vi "add_word.vi"(11 "子数组":u8[](array[numeric])) -> (3 "校验通过":bool)   [LabVIEW 2012]
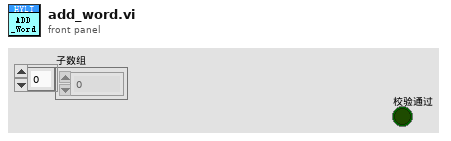
[diagram p1: front panel]
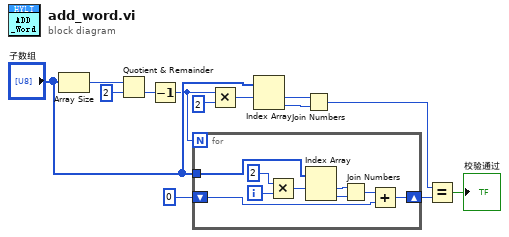
[diagram p0: block diagram]
diagram:
  n1 = Array Size(array="子数组") -> (size(s)=w11:i32)
  n2 = Quotient & Remainder(x=w11, y=2) -> (floor(x/y)=w6:i32)  [unwired: 1 out]
  n3 = Decrement(x=w6) -> (x-1=w3:i32)
  n4 = for {
    N: w3 -> [_]
    tunnel: "子数组" -> [w22]
    shift-right: [w14] -> w4
    shift-left: u16 0 -> [w15]
    i -> [w21]
    n5 = Multiply(x=2, y=w21) -> (x*y=w19:i32)
    n6 = Index Array(array=w22, index #1=w19) -> (element #1=w18:u8, element #2=w17:u8)  [unwired: 1 in]
    n7 = Join Numbers(hi=w18, lo=w17) -> ((hi.lo)=w16:u16)
    n8 = Add(x=w16, y=w15) -> (x+y=w14:u16)
  }
  n9 = Multiply(x=w3, y=2) -> (x*y=w1:i32)
  n10 = Index Array(array="子数组", index #1=w1) -> (element #1=w8:u8, element #2=w9:u8)  [unwired: 1 in]
  n11 = Join Numbers(hi=w8, lo=w9) -> ((hi.lo)=w5:u16)
  n12 = Equal?(x=w5, y=w4) -> (x = y?=→"校验通过":bool)
